vi "Import Spec From Excel.vi"(0 "Spec Path":path) -> (20 "Spec _Data":dbl[][](array[numeric]))   [LabVIEW 2011]
panel:
  in  "Excel._Worksheet":refnum<k7>
  in  "Excel._Application":refnum<k7>
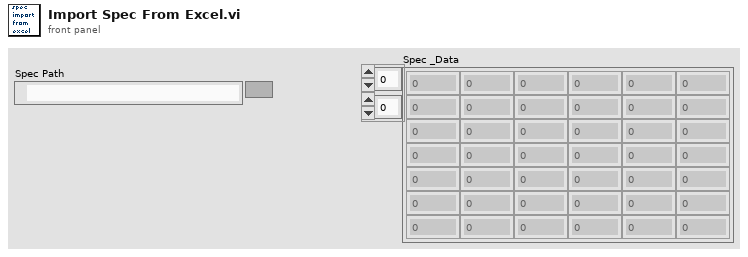
[diagram p1: front panel]
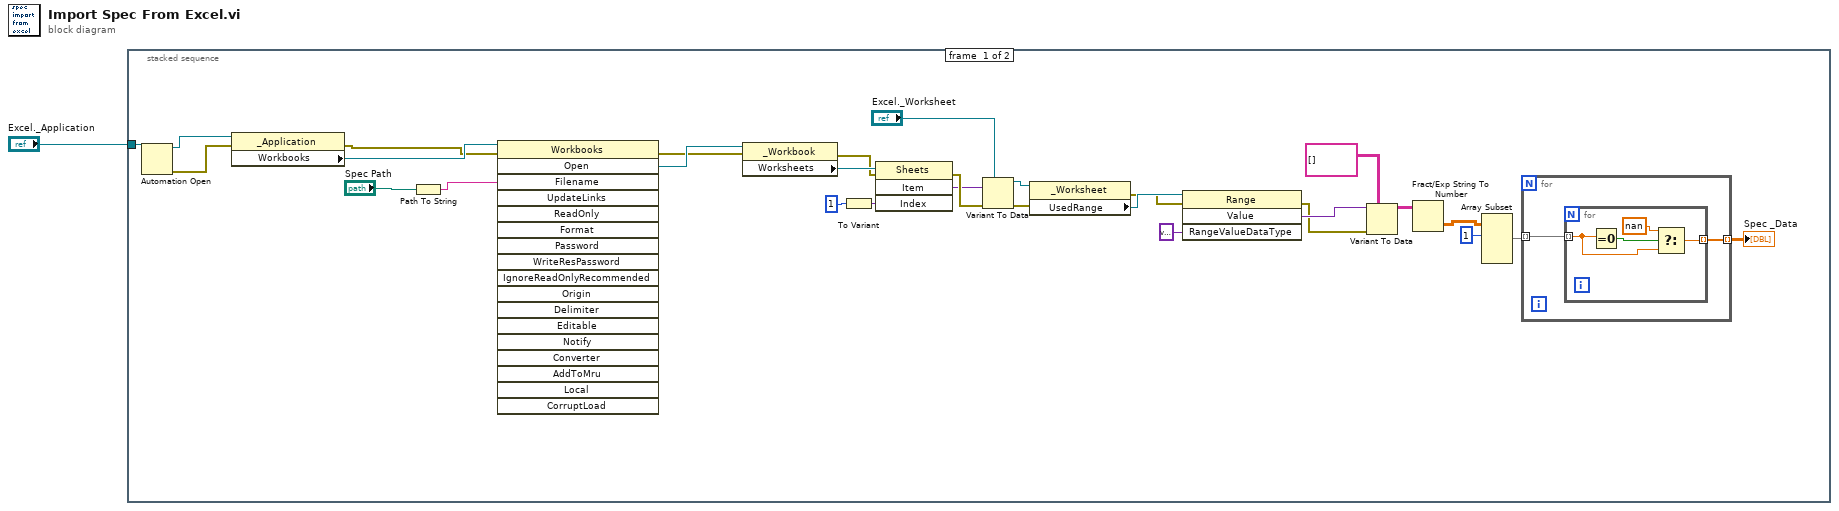
[diagram p0: block diagram]
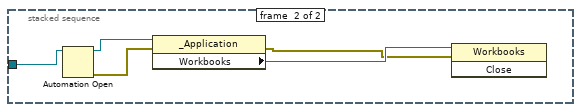
[diagram p2: hidden frame]
diagram:
  n1 = stacked-sequence {
    tunnel: "Excel._Application" -> [w30 w37]
    frame #0 {
      n2 = Automation Open(Automation Refnum=w30) -> (Automation Refnum=w29:refnum<k7>, error out=w28:errorcluster)  [unwired: 3 in]
      n3 = property class="_Application"(reference=w29, error in=w28) -> (error out=w26:errorcluster, "Workbooks"=w27:refnum<k7>)  [unwired: 1 out]
      n4 = Path To String(path="Spec Path") -> (string=w25:string)
      n5 = invoke class="Workbooks" method="Open"(reference=w27, error in=w26, "Filename"=w25) -> (error out=w22:errorcluster, "Open"=w23:refnum<k7>)  [unwired: 15 in, 16 out]
      n6 = property class="_Workbook"(reference=w23, error in=w22) -> (error out=w17:errorcluster, "Worksheets"=w21:refnum<k7>)  [unwired: 1 out]
      n7 = To Variant(anything=1) -> (Variant=w19:variant)
      n8 = invoke class="Sheets" method="Item"(reference=w21, error in=w17, "Index"=w19) -> (error out=w18:errorcluster, "Item"=w16:variant)  [unwired: 1 in, 2 out]
      n9 = Variant To Data(error in=w18, type="Excel._Worksheet", Variant=w16) -> (data=w14:refnum<k7>, error out=w13:errorcluster)
      n10 = property class="_Worksheet"(reference=w14, error in=w13) -> (error out=w9:errorcluster, "UsedRange"=w10:refnum<k7>)  [unwired: 1 out]
      n11 = invoke class="Range" method="Value"(reference=w10, error in=w9, "RangeValueDataType"=variant) -> (error out=w8:errorcluster, "Value"=w12:variant)  [unwired: 1 in, 2 out]
      n12 = Variant To Data(error in=w8, type=string[][] [] ("添加的数组"), Variant=w12) -> (data=w7:string[][])  [unwired: 1 out]
      n13 = Fract/Exp String To Number(string=w7) -> (number=w6:dbl[][])  [unwired: 3 in, 1 out]
      n14 = Array Subset(array=w6, index (row)=1 ("索引")) -> (w4:dbl[][])  [unwired: 3 in]
      n15 = for {
        tunnel: w4 -> [w32] mode=indexing
        tunnel: [w31] -> w3 mode=indexing
        n16 = for {
          tunnel: w32 -> [w34] mode=indexing
          tunnel: [w33] -> w31 mode=indexing
          n17 = Equal To 0?(x=w34) -> (x = 0?=w36:bool)
          n18 = Select(t=nan, s=w36, f=w34) -> (s? t:f=w33:dbl)
        }
      }
      "Spec _Data" <- w3
    }
    frame #1 {
      n19 = Automation Open(Automation Refnum=w37) -> (Automation Refnum=w41:refnum<k7>, error out=w40:errorcluster)  [unwired: 3 in]
      n20 = property class="_Application"(reference=w41, error in=w40) -> (error out=w38:errorcluster, "Workbooks"=w39:refnum<k7>)  [unwired: 1 out]
      n21 = invoke class="Workbooks" method="Close"(reference=w39, error in=w38) -> ()  [unwired: 1 in, 3 out]
    }
  }
